vi "solar_write UnsubscribeThisUE.vi"(8 "error in (no error)":errorcluster, 10 "Destination Target":string, 11 "solar in":refnum<class "solar.lvclass">) -> (0 "error out":errorcluster, 3 "solar out":refnum<class "solar.lvclass">)   [LabVIEW 2018, in "solar.lvclass"]
doc: "This unsubscribes this target's user event from the distination target. (i.e. Stops the destination target from relaying telemetry to this target)"
uses:
  solar.lvclass
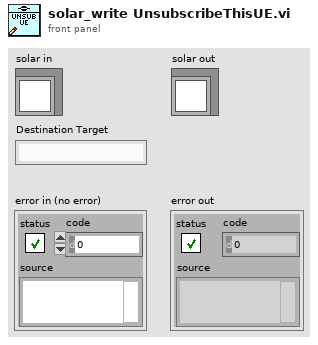
[diagram p1: front panel]
types:
  T1 = typedef "solar_ctl SOLAR Refnum.ctl" = refnum<k1>
  T2 = typedef "solar_ctl SOLAR Global.ctl" = cluster{"Targets":T3[], "AppDir":path, "solar.ini":path, "ConfigsDir":path, "CosmosDir":path, "LogsDir":path, "ExePath":path, "ExeVersion":string, "PartNum":string, "AppSetup":string, "Title":string, "Main.ini":path, "Temp.ini":path, "vSOLAR":string, "Splash.png":string, "SplashWait":i32, "SOLARUE":refnum<user-event>, "VoyagerRefnum":T4, "QTimerRefnum":T5}
  T3 = typedef "solar_ctl Target Global.ctl" = cluster{"Target":string, "Q":refnum<queue>, "UE":refnum<user-event>, "VI":refnum<vi>, "Menu":refnum<k9>, "Data":refnum<data-value>, "Attributes":variant}
  T4 = typedef "solar_voy_ctl Voyager Refnum.ctl" = refnum<k1>
  T5 = typedef "solar_qtimer_ctl Refnum.ctl" = refnum<k1>
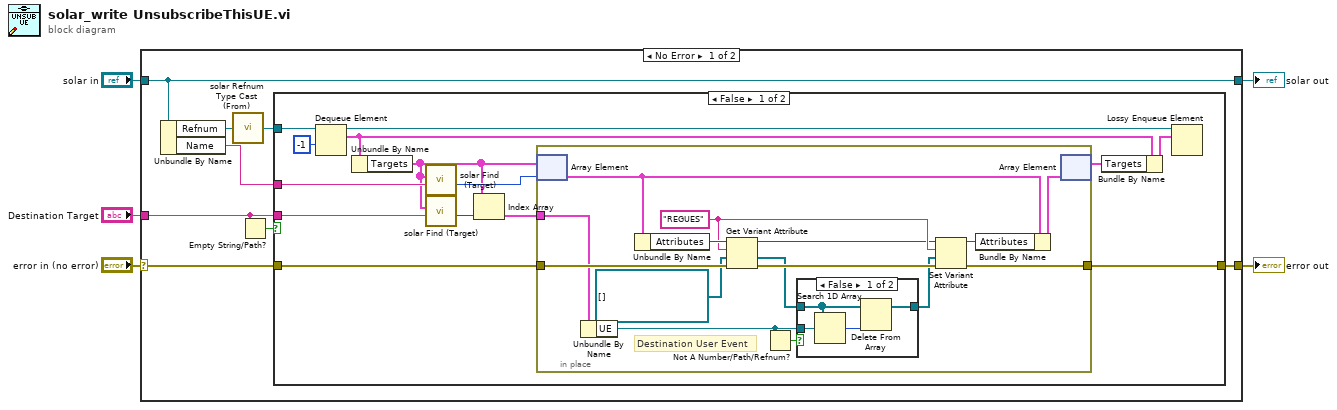
[diagram p0: block diagram]
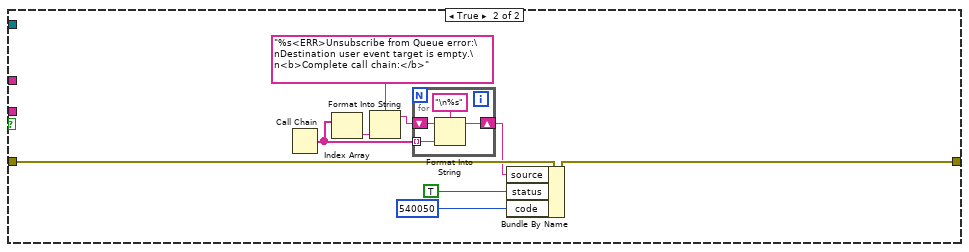
[diagram p3: hidden frame]
diagram:
  n1 = case shown="No Error" "error in (no error)" {
    selector: "error in (no error)" -> [w12 w62]
    tunnel: "solar in" -> [w13 w61]
    tunnel: [w9 w62] -> w1
    tunnel: [w13 w61] -> w2
    tunnel: "Destination Target" -> [w7 _]
    frame No Error {
      n2 = Unbundle By Name(w13) -> ("Refnum"=w11:T1, "Name"=w8:string)
      n3 = call "solar Refnum Type Cast (From).vi"("Refnum"=w11) -> ("SOLAR"=w10:refnum<queue>)
      n4 = Empty String/Path?(string/path=w7) -> (empty?=w6:bool)
      n5 = case shown="False" w6 {
        tunnel: w12 -> [w27 w50]
        tunnel: w10 -> [w26 _]
        tunnel: [w23 w48] -> w9
        tunnel: w8 -> [w20 _]
        tunnel: w7 -> [w19 _]
        frame False {
          n6 = Dequeue Element(queue=w26, timeout in ms (-1)=-1) -> (queue out=w25:refnum<queue>, element=w22:T2)  [unwired: 1 in, 2 out]
          n7 = Unbundle By Name(w22) -> ("Targets"=w16:T3[])
          n8 = call "solar Find (Target).vi"("Target"=w20, "Targets"=w16) -> ("Target Index"=w18:i32)  [unwired: 8 in, 1 out]
          n9 = call "solar Find (Target).vi"("Target"=w19, "Targets"=w16) -> ("Target Index"=w15:i32)  [unwired: 8 in, 1 out]
          n10 = Index Array(array=w16, index=w15) -> (element=w14:T3)
          n11 = in-place {
            in-place-border: w27 -> [w39]
            in-place-border: [w38] -> w23
            in-place-border: w14 -> [w28]
            w35 = "REGUES" ("name")
            # "Destination User Event"
            n12 = in-place-array #1(w16, w18) -> (w42:T3)
            n13 = Unbundle By Name(w28) -> ("UE"=w30:refnum<user-event>)
            n14 = Unbundle By Name(w42) -> ("Attributes"=w36:variant)
            n15 = Get Variant Attribute(Variant=w36, name=w35, default value (empty Variant)=refnum<user-event>[] [] ("RegUEs"), error in=w39) -> (duplicate Variant=w34:variant, value=w32:refnum<user-event>[], error out=w37:errorcluster)  [unwired: 1 out]
            n16 = Not A Number/Path/Refnum?(number/path/refnum=w30) -> (NaN/Path/Refnum?=w33:bool)
            n17 = case shown="False" w33 {
              tunnel: w32 -> [w45 w47]
              tunnel: [w43 w47] -> w31
              tunnel: w30 -> [w46 _]
              frame False {
                n18 = Search 1D Array(1D array=w45, element=w46) -> (index of element=w44:i32)  [unwired: 1 in]
                n19 = Delete From Array(array=w45, index=w44) -> (array with subset deleted=w43:refnum<user-event>[])  [unwired: 1 in, 1 out]
              }
              frame True {
              }
            }
            n20 = Set Variant Attribute(Variant=w34, name=w35, value=w31, error in=w37) -> (Variant out=w40:variant, error out=w38:errorcluster)  [unwired: 1 out]
            n21 = Bundle By Name(cluster=w42, "Attributes"=w40) -> (w41:T3)
            n22 = in-place-array #1(w41) -> (w17:T3[])  [unwired: 1 out]
          }
          n23 = Bundle By Name(cluster=w22, "Targets"=w17) -> (w21:T2)
          n24 = Lossy Enqueue Element(queue=w25, element=w21) -> ()  [unwired: 1 in, 4 out]
        }
        frame True {
          n25 = Call Chain() -> (call chain=w51:string[])
          n26 = Index Array(array=w51) -> (element=w53:string)  [unwired: 1 in]
          n27 = Format Into String(format string="%s<ERR>Unsubscribe from Queue error:\nDestination user event target is empty.\n<b>Complete call chain:</b>", w53) -> (resulting string=w52:string)  [unwired: 2 in, 1 out]
          n28 = for {
            tunnel: w51 -> [w60] mode=indexing
            shift-right: [w59] -> w49
            shift-left: w52 -> [w58]
            n29 = Format Into String(format string="\n%s", initial string=w58, w60) -> (resulting string=w59:string)  [unwired: 1 in, 1 out]
          }
          n30 = Bundle By Name(cluster=w50, "source"=w49, "status"=TRUE, "code"=540050 ("Code")) -> (w48:errorcluster)
        }
      }
    }
    frame Error {
    }
  }
  "error out" <- w1
  "solar out" <- w2
